vi "Simple Single Point Benchmark.vi"() -> ()   [LabVIEW 2011]
uses:
  <instrlib>/niDMM/nidmm.llb/niDMM Function.ctl
  <instrlib>/niDMM/nidmm.llb/niDMM Auto Zero.ctl
  <instrlib>/niDMM/nidmm.llb/niDMM ADC Calibration.ctl
  <instrlib>/niDMM/nidmm.llb/niDMM Configure Measurement Absolute.vi
panel:
  in  "Resolution":dbl=1e-05 format="%.5f"
  out "Measurement Period (seconds)":dbl format="%.4f"
  in  "ADC Calibration":T1=-1 items=["Auto"=-1, "Off"=0, "On"=1]
  in  "Auto Zero":T2=1 items=["Auto"=-1, "Off"=0, "On"=1, "Once"=2]
  in  "Range":dbl=10.0 format="%.2f"
  in  "Function":T3
  in  "Instrument Descriptor":refnum<k15>="DMM"
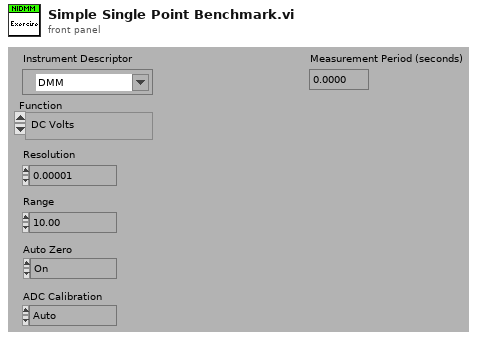
[diagram p1: front panel]
types:
  T1 = typedef "niDMM ADC Calibration.ctl" = i32
  T2 = typedef "niDMM Auto Zero.ctl" = i32
  T3 = typedef "niDMM Function.ctl" = enum16{"DC Volts", "AC Volts", "DC Current", "AC Current", "2-wire Resistance", "4-wire Resistance", "Diode", "Frequency", "Period", "AC Volts DC Coupled", "Capacitance", "Inductance", "Temperature"}
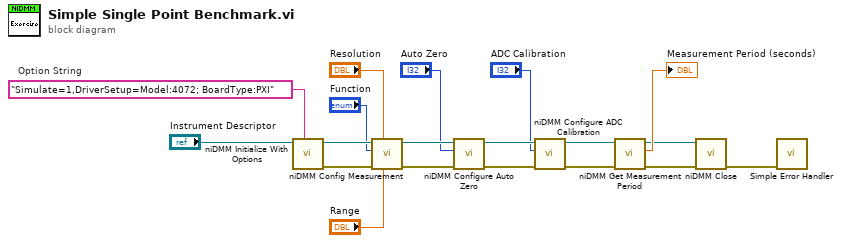
[diagram p0: block diagram]
diagram:
  w1 = "Simulate=1,DriverSetup=Model:4072; BoardType:PXI"  # Option String
  n1 = call <instrlib>:"niDMM Initialize With Options.vi"("Option String"=w1, "Instrument Descriptor"="Instrument Descriptor") -> ("error out"=w17:errorcluster, "instrument handle out"=w18:refnum<k15>)  [unwired: 8 in]
  n2 = call-poly <instrlib>:"niDMM Config Measurement.vi"("Range"="Range", "Resolution"="Resolution", "error in (no error)"=w17, "Function"="Function", "instrument handle"=w18) -> ("error out"=w13:errorcluster, "instrument handle out"=w14:refnum<k15>)  [unwired: 5 in]
  n3 = call <instrlib>:"niDMM Configure Auto Zero.vi"("error in (no error)"=w13, "Auto Zero"="Auto Zero", "instrument handle"=w14) -> ("error out"=w10:errorcluster, "instrument handle out"=w11:refnum<k15>)  [unwired: 7 in]
  n4 = call <instrlib>:"niDMM Configure ADC Calibration.vi"("error in (no error)"=w10, "ADC Calibration"="ADC Calibration", "instrument handle"=w11) -> ("error out"=w8:errorcluster, "instrument handle out"=w7:refnum<k15>)  [unwired: 7 in]
  n5 = call <instrlib>:"niDMM Get Measurement Period.vi"("error in (no error)"=w8, "instrument handle"=w7) -> ("error out"=w5:errorcluster, "Measurement Period (seconds)"=→"Measurement Period (seconds)":dbl, "instrument handle out"=w4:refnum<k15>)  [unwired: 7 in]
  n6 = call <instrlib>:"niDMM Close.vi"("error in (no error)"=w5, "instrument handle"=w4) -> ("error out"=w3:errorcluster)  [unwired: 9 in]
  n7 = call <vilib>:"Simple Error Handler.vi"("error in (no error)"=w3) -> ()  [unwired: 4 in, 5 out]
